vi "GLdrv_ANN.vi"(0 "Connection ID":T1, 5 "CH":i32=1 min=1, 7 "Annotation":string, 11 "error in (no error)":errorcluster, 13 "Query(f)":bool) -> (4 "Connection ID Out":T1, 8 "Annotation out":string, 15 "error out":errorcluster)   [LabVIEW 2017, in "GL860_Driver.lvlib"]
doc: "アノテーションの設定・参照\n最大文字数31文字,英数半角ｶﾅが入力可能です。\n例) ANN:CH5 “SOKUTEI” (CH5のアノテーションを”SOKUTEI”\nに設定します)"
uses:
  GL860_Driver.lvlib
  ConnectionID.ctl
  GLdrv_RW.ctl
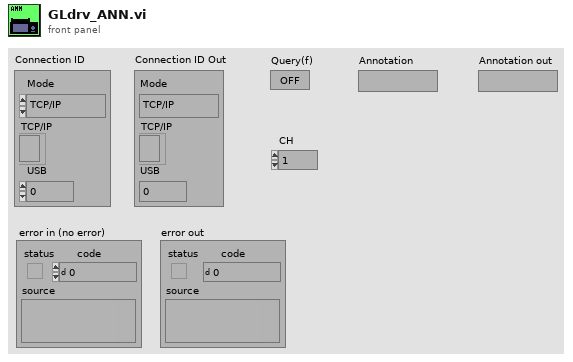
[diagram p1: front panel]
types:
  T1 = typedef "ConnectionID.ctl" = cluster{"Mode":enum16{"TCP/IP", "USB"}, "TCP/IP":refnum<k5>, "USB":i32}
  T2 = typedef "GLdrv_RW.ctl" = enum16{"Auto", "Read", "Write", "Buffer"}
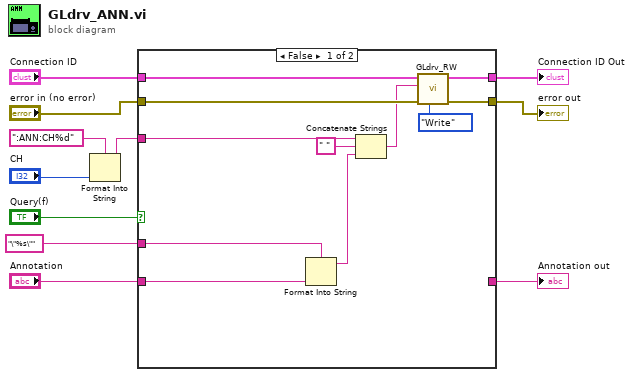
[diagram p0: block diagram]
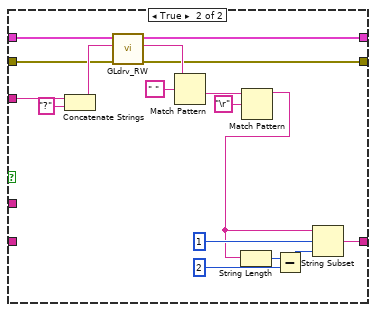
[diagram p2: hidden frame]
diagram:
  n1 = Format Into String(format string=":ANN:CH%d" ("Command"), "CH") -> (resulting string=w5:string)  [unwired: 2 in, 1 out]
  n2 = case shown="FALSE" "Query(f)" {
    tunnel: w5 -> [w22 w36]
    tunnel: [w17 w29] -> w11
    tunnel: [w19 w33] -> w10
    tunnel: "Connection ID" -> [w20 w34]
    tunnel: "error in (no error)" -> [w18 w30]
    tunnel: "Annotation" -> [w13 _]
    tunnel: [_ w24] -> w2
    tunnel: "\"%s\"" ("Param") -> [w12 _]
    frame False {
      n3 = Format Into String(format string=w12, w13) -> (resulting string=w14:string)  [unwired: 2 in, 1 out]
      n4 = Concatenate Strings(w22, " " ("string"), w14) -> (w16:string)
      n5 = call "GLdrv_RW.vi"("Mode(read)"=GLdrv_RW."Write", "error in (no error)"=w18, "data in"=w16, "Connection ID"=w20) -> ("error out"=w17:errorcluster, "Connection ID Out"=w19:T1)  [unwired: 3 in, 3 out]
    }
    frame True {
      n6 = Concatenate Strings(w36, "?" ("string")) -> (w32:string)
      n7 = call "GLdrv_RW.vi"("error in (no error)"=w30, "data in"=w32, "Connection ID"=w34) -> ("error out"=w29:errorcluster, "data out"=w31:string, "Connection ID Out"=w33:T1)  [unwired: 4 in, 2 out]
      n8 = Match Pattern(string=w31, regular expression=" " ("search string/char (-)")) -> (after substring=w37:string)  [unwired: 4 out]
      n9 = Match Pattern(string=w37, regular expression="\r") -> (before substring=w23:string)  [unwired: 4 out]
      n10 = String Length(string=w23) -> (length=w27:i32)
      n11 = Subtract(x=w27, y=2) -> (x-y=w26:i32)
      n12 = String Subset(string=w23, offset (0)=1, length (rest)=w26) -> (substring=w24:string)
    }
  }
  "Connection ID Out" <- w10
  "error out" <- w11
  "Annotation out" <- w2
